vi "VIPCApply.vi"() -> ()   [LabVIEW 2011, in "G CLI VIP.lvlib"]
uses:
  G CLI VIP.lvlib
  <vilib>/Wiresmith Technology/G CLI/CLI Class/CLI.lvclass
  <vilib>/JKI/VIPM API/VIPM API_vipm_api.lvlib
panel:
  out "error out":errorcluster
  # "VIPC Apply"
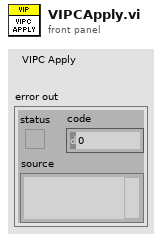
[diagram p1: front panel]
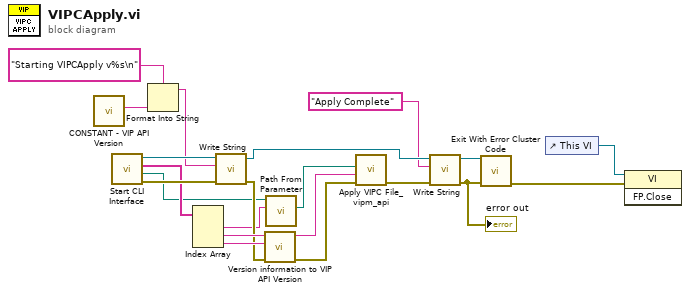
[diagram p0: block diagram]
diagram:
  n1 = call "CONSTANT - VIP API Version.vi"() -> ("Version"=w18:string)  [unwired: 11 in]
  n2 = call <vilib>:"Start CLI Interface.vi"() -> ("error out"=w20:errorcluster, "Working Directory"=w8:path, "Custom Parameters"=w15:string[], "CLI out"=w21:refnum<class "CLI.lvclass">)  [unwired: 8 in]
  n3 = Format Into String(format string="Starting VIPCApply v%s\n", w18) -> (resulting string=w17:string)  [unwired: 2 in, 1 out]
  n4 = Index Array(array=w15) -> (element #1=w9:string, element #2=w14:string, element #3=w13:string)  [unwired: 3 in]
  n5 = call <vilib>:"Write String.vi"("error in (no error)"=w20, "Text to Write"=w17, "CLI in"=w21) -> ("error out"=w12:errorcluster, "CLI out"=w4:refnum<class "CLI.lvclass">)  [unwired: 7 in]
  n6 = call "Version information to VIP API Version.vi"("error in (no error)"=w12, "Bitness String"=w13, "Version String"=w14) -> ("error out"=w11:errorcluster, "VIP Version"=w10:string)  [unwired: 7 in]
  n7 = call <vilib>:"Path From Parameter.vi"("Path Parameter"=w9, "Working Directory"=w8) -> ("Full Path"=w7:path)  [unwired: 9 in]
  n8 = call <vilib>:"Apply VIPC File_vipm_api.vi"("error in (no error)"=w11, "LabVIEW Version"=w10, "VIPC File"=w7) -> ("error out"=w16:errorcluster)  [unwired: 8 in]
  n9 = call <vilib>:"Write String.vi"("error in (no error)"=w16, "Text to Write"="Apply Complete", "CLI in"=w4) -> ("error out"=w6:errorcluster, "CLI out"=w5:refnum<class "CLI.lvclass">)  [unwired: 7 in]
  "error out" <- w6
  n10 = call <vilib>:"Exit With Error Cluster Code.vi"("error in (no error)"=w6, "CLI in"=w5) -> ("error out"=w2:errorcluster)  [unwired: 9 in]
  n11 = control-ref of="This VI"() -> (w1:refnum<vi>)
  n12 = invoke class="VI" method="FP.Close"(reference=w1, error in=w2) -> ()  [unwired: 1 in, 3 out]
